vi "Create_Waveform.vi"(10 "Array":u8[](array[numeric]), 11 "Sample Rate [S/s]":dbl=1.0) -> (3 "output waveform":waveform(u8))   [LabVIEW 2016]
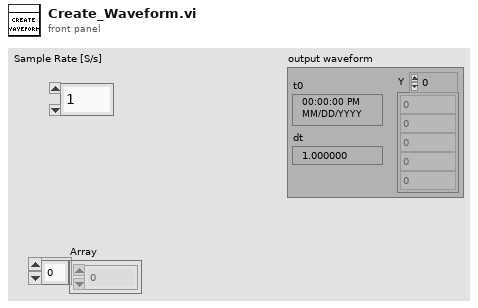
[diagram p1: front panel]
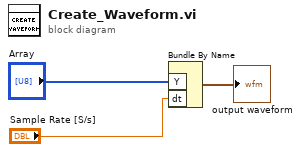
[diagram p0: block diagram]
diagram:
  n1 = Bundle By Name("Y"="Array", "dt"="Sample Rate [S/s]") -> (→"output waveform":waveform(u8))  [unwired: 1 in]
